vi "Check If Aligned to 8-byte Boundary.vi"(11 "pointer":u32 format="%08x") -> (2 "aligned?":bool, 3 "pointer out":u32 format="%08x")   [LabVIEW 2016, in "GE 5565PIORC.lvclass"]
uses:
  GE 5565PIORC.lvclass
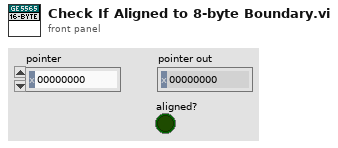
[diagram p1: front panel]
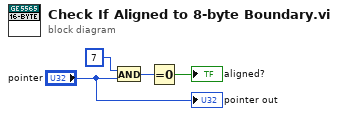
[diagram p0: block diagram]
diagram:
  n1 = And(x=u32 7, y="pointer") -> (x .and. y?=w3:u32)
  n2 = Equal To 0?(x=w3) -> (x = 0?=→"aligned?":bool)
  "pointer out" <- "pointer"
